vi "newTemp.vi"(11 "port":u16=3000) -> (3 "Response String":string)   [LabVIEW 2018]
uses:
  <vilib>/Utility/error.llb/DialogType.ctl
  <vilib>/regexp/Match Regular Expression.xnode
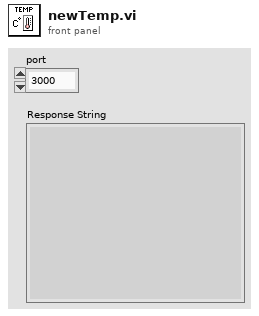
[diagram p1: front panel]
types:
  T1 = typedef "DialogType.ctl" = u16
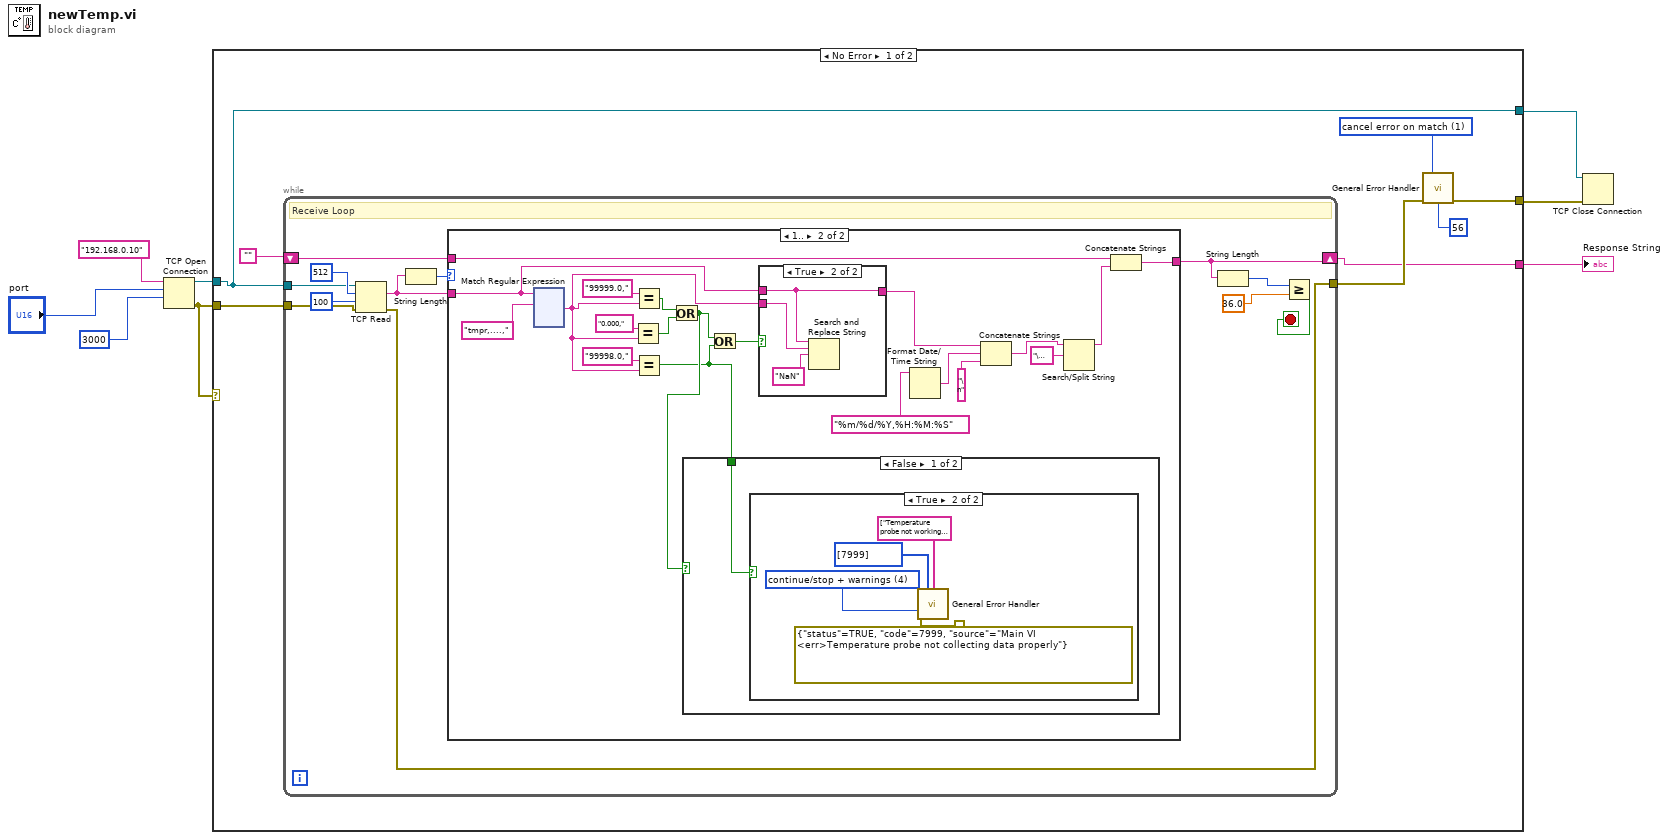
[diagram p0: block diagram]
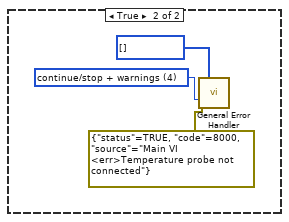
[diagram p4: hidden frame]
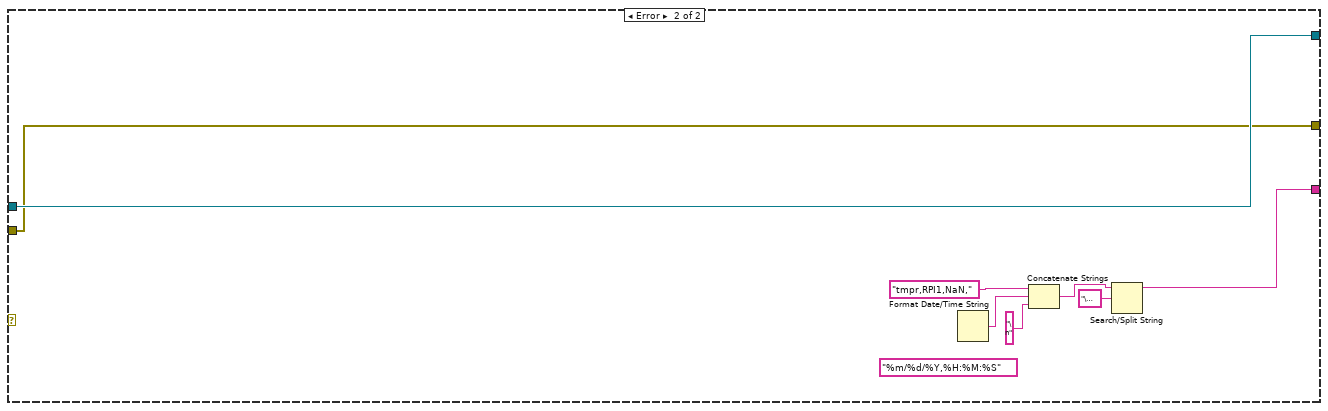
[diagram p6: hidden frame]
diagram:
  n1 = TCP Open Connection(address="192.168.0.10", remote port or service name="port", timeout ms (60000)=3000) -> (connection ID=w3:refnum<k5>, error out=w4:errorcluster)  [unwired: 2 in]
  n2 = case shown="No Error" w4 {
    tunnel: [w10 w176] -> w1
    tunnel: w3 -> [w14 w183]
    tunnel: w4 -> [w15 w176]
    tunnel: [w14 w183] -> w5
    tunnel: [w9 w177] -> w2
    frame No Error {
      w13 = 1 items=["no exception", "cancel error on match", "set error on match"] ("[exception action] (none:0)")
      n3 = while "Receive loop" {
        shift-left: "" -> [w26]
        shift-right: [w18] -> w9
        tunnel: [w21] -> w11
        tunnel: w14 -> [w23]
        tunnel: w15 -> [w22]
        stop <- w17 stop-if-true
        # "Receive Loop"
        n4 = TCP Read(connection ID=w23, bytes to read=512, error in (no error)=w22, 9:100) -> (data out=w25:string, error out=w21:errorcluster)  [unwired: 1 in, 1 out]
        n5 = String Length(string=w25) -> (length=w28:i32)
        n6 = case shown="1.." w28 {
          tunnel: w25 -> [_ w42]
          tunnel: w26 -> [w29 w33]
          tunnel: [w29 w32] -> w18
          frame ..0 {
          }
          frame 1.. {
            n7 = xnode "Match Regular Expression"("input string"=w42, "regular expression"="tmpr,....,") -> ("after match"=w41:string)  [unwired: 4 in, 4 out]
            n8 = Equal?(x="0.000,", y=w41) -> (x = y?=w44:bool)
            n9 = Equal?(x="99999.0," ("y"), y=w41) -> (x = y?=w45:bool)
            n10 = Equal?(x="99998.0," ("y"), y=w41) -> (x = y?=w30:bool)
            n11 = Or(x=w45, y=w44) -> (x .or. y?=w31:bool)
            n12 = case shown="False" w31 {
              tunnel: w30 -> [w50 _]
              frame False {
                n13 = case shown="True" w50 {
                  frame False {
                  }
                  frame True {
                    w52 = T1 4 items=["no dialog", "OK message", "continue or stop message", "OK message + warnings", "continue/stop + warnings"] ("type of dialog (OK msg:1)")
                    n14 = call <vilib>:"General Error Handler.vi"("[user-defined codes]"=i32[] [7999], "[user-defined descriptions]"=string[] ["Temperature probe not working properly"], "type of dialog (OK msg:1)"=w52, "error in (no error)"=errorcluster {"status"=TRUE, "code"=7999, "source"="Main VI <err>Temperature probe not collecting data properly"}) -> ()  [unwired: 7 in, 5 out]
                  }
                }
              }
              frame True {
                w56 = T1 4 items=["no dialog", "OK message", "continue or stop message", "OK message + warnings", "continue/stop + warnings"] ("type of dialog (OK msg:1)")
                n15 = call <vilib>:"General Error Handler.vi"("[user-defined codes]"=i32[] [], "type of dialog (OK msg:1)"=w56, "error in (no error)"=errorcluster {"status"=TRUE, "code"=8000, "source"="Main VI <err>Temperature probe not connected"}) -> ()  [unwired: 8 in, 5 out]
              }
            }
            n16 = Or(x=w31, y=w30) -> (x .or. y?=w43:bool)
            n17 = case shown="True" w43 {
              tunnel: w42 -> [w58 w59]
              tunnel: w41 -> [_ w61]
              tunnel: [w58 w59] -> w40
              frame False {
              }
              frame True {
                n18 = Search and Replace String(input string=w59, search string=w61, replace string="NaN" ("replace string (\"\")")) -> ()  [unwired: 5 in, 4 out]
              }
            }
            n19 = Format Date/Time String(time format string (%c)="%m/%d/%Y,%H:%M:%S") -> (date/time string=w38:string)  [unwired: 2 in]
            n20 = Concatenate Strings(w40, w38, "\n" ("string")) -> (w36:string)
            n21 = Search/Split String(string=w36, search string/char (-)="\u0004") -> (substring before match=w34:string)  [unwired: 1 in, 2 out]
            n22 = Concatenate Strings(w33, w34) -> (w32:string)
          }
        }
        n23 = String Length(string=w18) -> (length=w20:i32)
        n24 = Greater Or Equal?(x=w20, y=36.0) -> (x >= y?=w17:bool)
      }
      n25 = call <vilib>:"General Error Handler.vi"("error in (no error)"=w11, "[exception action] (none:0)"=w13, "[exception code]"=56) -> ("error out"=w10:errorcluster)  [unwired: 8 in, 4 out]
    }
    frame Error {
      (unwired) "%m/%d/%Y,%H:%M:%S" ("time format string (%c)")
      n26 = Format Date/Time String() -> (date/time string=w180:string)  [unwired: 3 in]
      n27 = Concatenate Strings("tmpr,RPI1,NaN," ("string"), w180, "\n" ("string")) -> (w178:string)
      n28 = Search/Split String(string=w178, search string/char (-)="\u0004") -> (substring before match=w177:string)  [unwired: 1 in, 2 out]
    }
  }
  "Response String" <- w2
  n29 = TCP Close Connection(connection ID=w5, error in (no error)=w1) -> ()  [unwired: 1 in, 2 out]
